vi "Measurement selected.vi"(8 "error in (no error)":errorcluster, 10 "Coords":T1, 11 "ZenGage v3.0 UI in":T2) -> (0 "error out":errorcluster, 3 "ZenGage v3.0 UI in":T2)   [LabVIEW 2019, in "ZenGage v3.0 UI.lvclass"]
uses:
  ZenGage v3.0 UI.lvclass
  <vilib>/Utility/miscctls.llb/LVPoint32TypeDef.ctl
  Type Definitions/JSON Read/UI JSON read cluster.ctl
  Type Definitions/General/JSONRead.ctl
  Type Definitions/Inspection/Inspection Cluster.ctl
  Type Definitions/Diagnostics/Diagnostics(Cluster).ctl
  Type Definitions/Edit tolerance settings/Rack Selection.ctl
  Type Definitions/Edit tolerance settings/Edit Tolerance Input.ctl
  Type Definitions/Edit tolerance settings/Edit Tolerance Overall Cluster.ctl
  Type Definitions/Controls and Indicators/Select a part (combobox).ctl
  Type Definitions/Controls and Indicators/EDL control references.ctl
  Type Definitions/Controls and Indicators/Diagnostics control referencs.ctl
  Type Definitions/Controls and Indicators/Inspection control references.ctl
  Type Definitions/Controls and Indicators/General_Control references.ctl
  Type Definitions/Controls and Indicators/Controls and Indicators Cluster.ctl
  Common/Controls/Pop-up Input.ctl
  Type Definitions/General/UI States(UI button enable disable).ctl
  Type Definitions/General/UIDataCluster.ctl
  Type Definitions/General/Master sample references.ctl
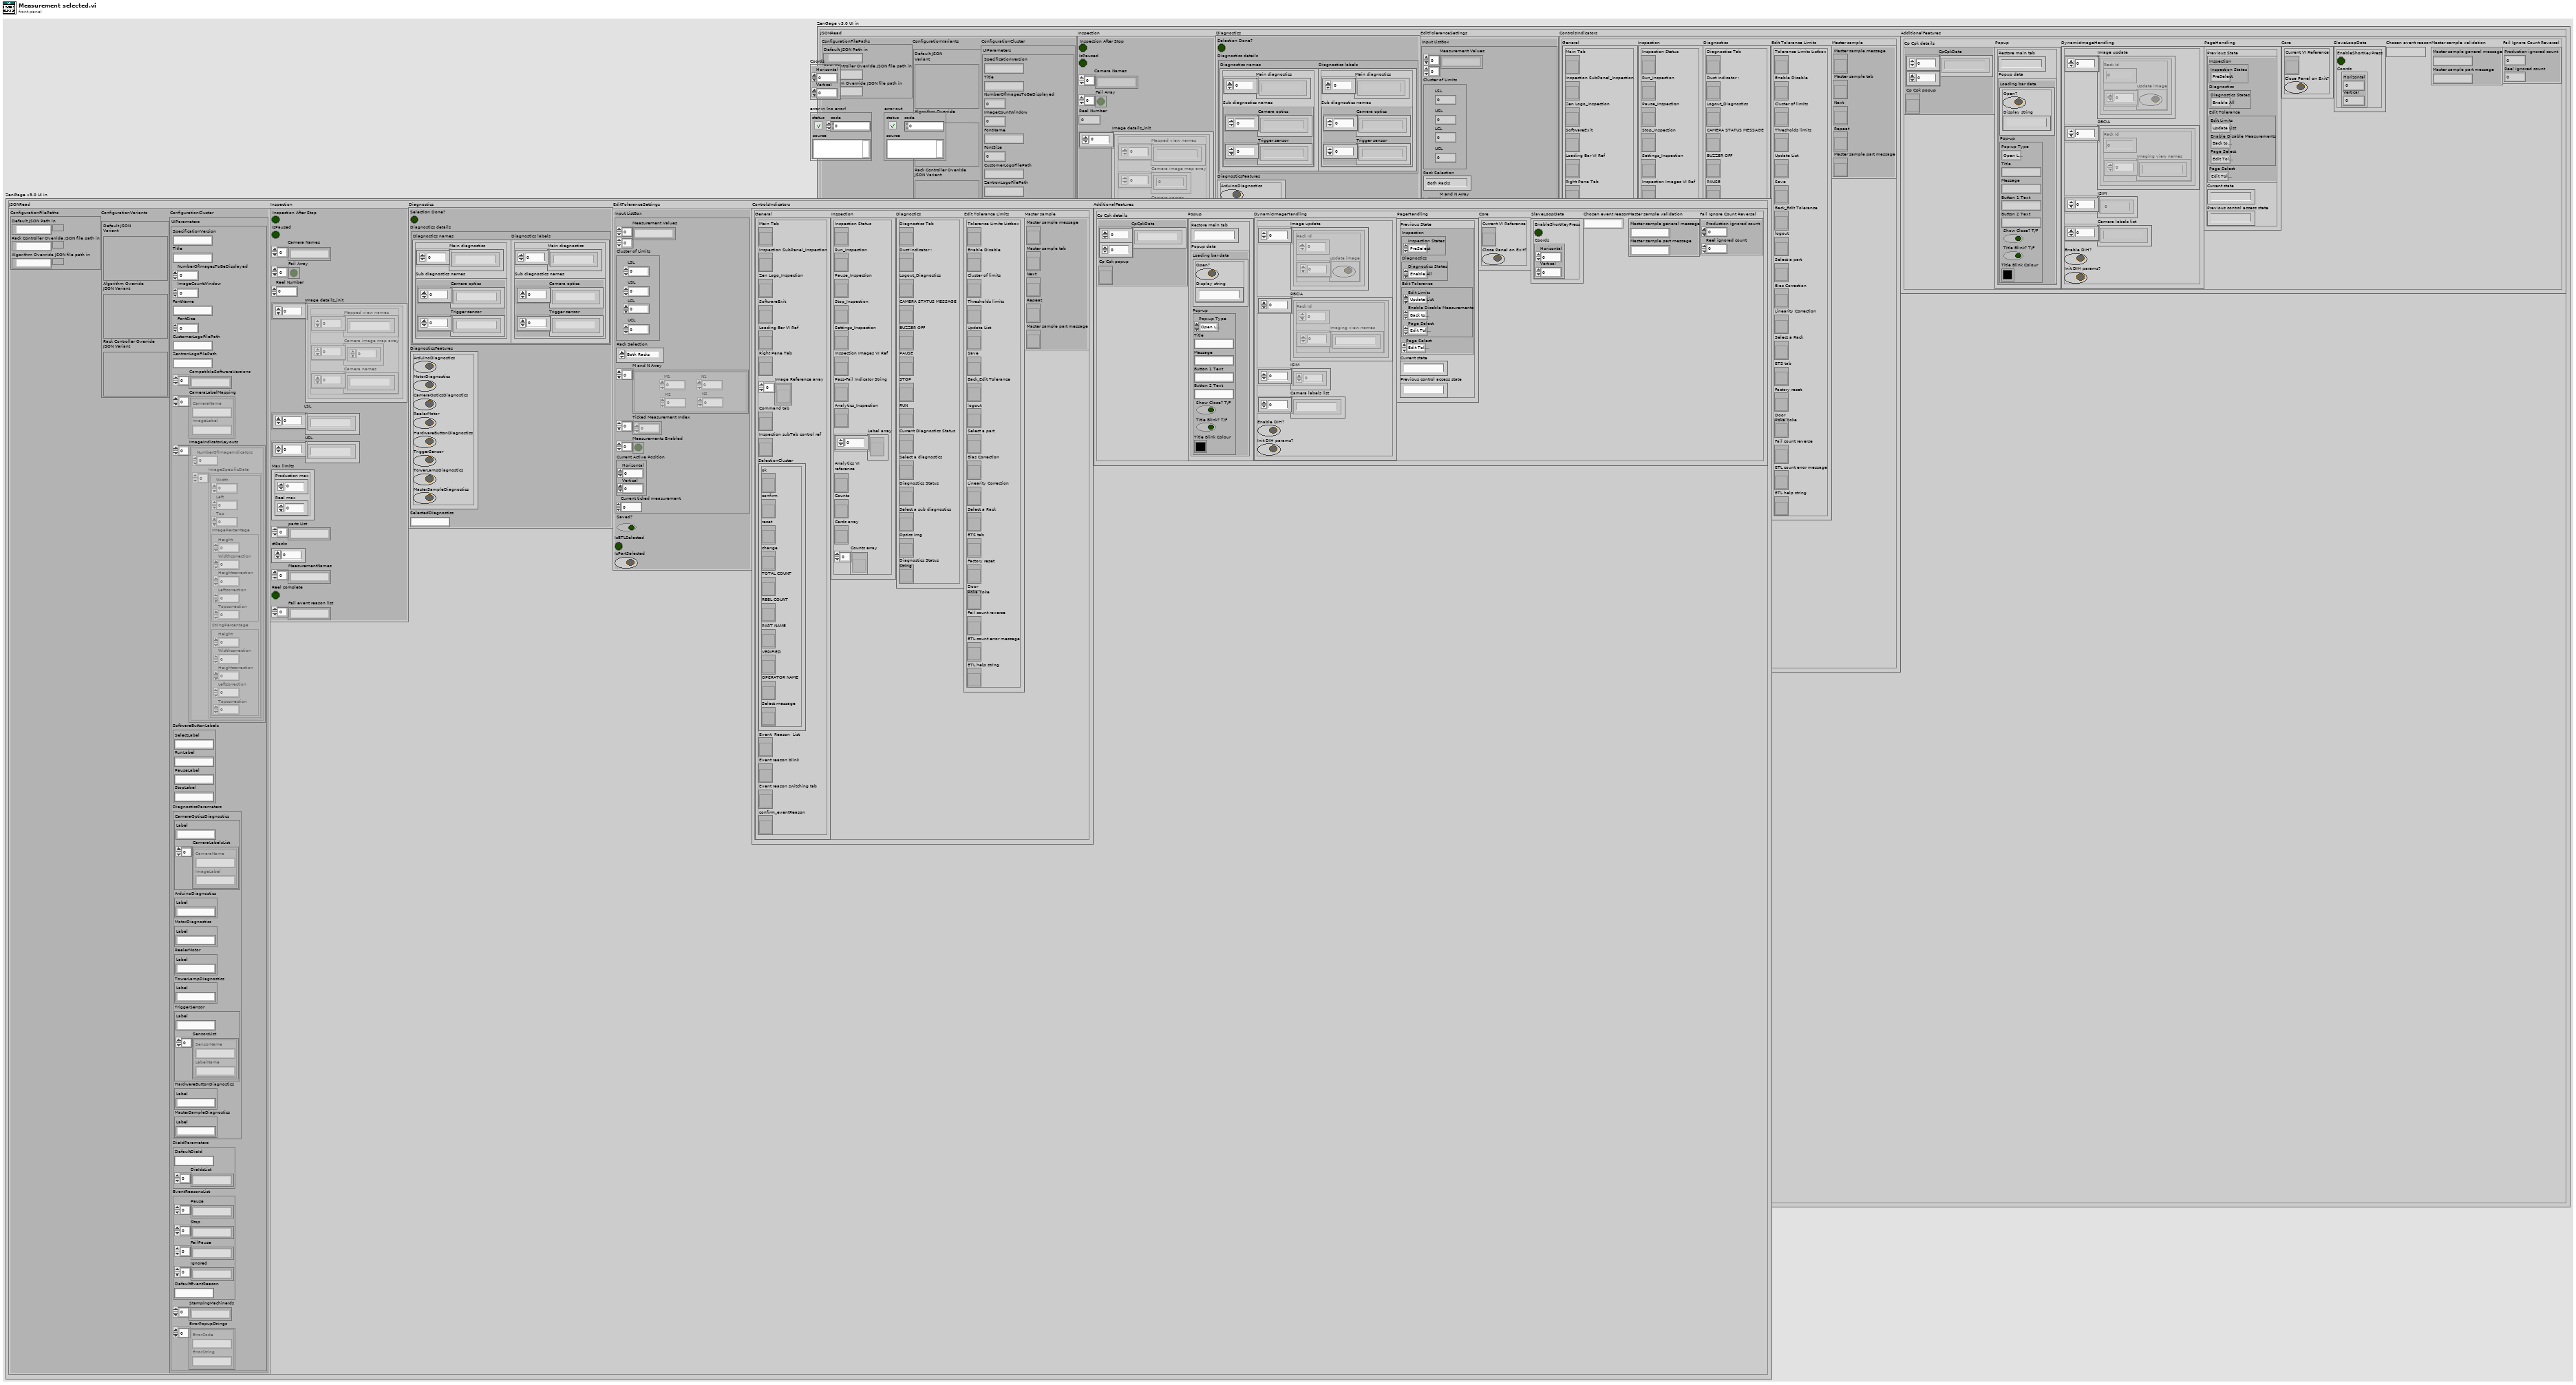
[diagram p1: front panel]
types:
  T1 = typedef "LVPoint32TypeDef.ctl" = cluster{"Horizontal":i32, "Vertical":i32}
  T2 = typedef "UIDataCluster.ctl" = cluster{"JSONRead":T3, "Inspection":T5, "Diagnostics":T6, "EditToleranceSettings":T7, "ControlsIndicators":T10, "AdditionalFeatures":cluster{"Cp Cpk details":cluster{"CpCpkData":string[][], "Cp Cpk popup":refnum<vi>}, "Popup":cluster{"Restore main tab":string, "Popup data":cluster{"Loading bar data":cluster{"Open?":bool, "Display string":string}, "Pop-up":T16}}, "DynamicImageHandling":cluster{"Image update":cluster{"Rack Id":i32, "Update image":bool[]}[], "RBCIA":cluster{"Rack Id":u8, "Imaging view names":string[]}[], "ISIM":u8[], "Camera labels list":string[], "Enable DIH?":bool, "Init DIH params?":bool}, "PageHandling":cluster{"Previous State":T17, "Current state":string, "Previous control access state":string}, "Core":cluster{"Current VI Reference":refnum<vi>, "Close Panel on Exit?":bool}, "SlaveLoopData":cluster{"EnableShortKeyPress":bool, "Point32":T1}, "Chosen event reason":string, "Master sample validation":cluster{"Master sample general message":string, "Master sample part message":string}, "Fail Ignore Count Reversal":cluster{"Production ignored count":u64, "Reel ignored count":u64}}}
  T3 = typedef "ZenGage v3.0 UI.lvclass/JSONRead.ctl" = cluster{"ConfigurationFilePaths":cluster{"Default JSON Path in":path, "Rack Controller Override JSON file path in":path, "Algorithm Overrride JSON file path in ":path}, "ConfigurationVariants":cluster{"Default JSON \nVariant":variant, "Algorithm Override\nJSON Variant":variant, "Rack Controller Override\nJSON Variant":variant}, "ConfigurationCluster":T4}
  T4 = typedef "ZenGage v3.0 UI.lvclass/UI JSON read cluster.ctl" = cluster{"UIParameters":cluster{"SpecificationVersion":string, "Title":string, "NumberOfImagesToBeDisplayed":dbl, "ImageCountWindow":dbl, "FontName":string, "FontSize":dbl, "CustomerLogoFilePath":string, "ZentronLogoFilePath":string, "CompatibleSoftwareVersions":string[], "CameraLabelMapping":cluster{"CameraName":string, "ImageLabel":string}[], "ImageIndicatorLayouts":cluster{"NumberOfImageIndicators":dbl, "ImageSpecificData":cluster{"Width":dbl, "Left":dbl, "Top":dbl, "ImagePercentage":cluster{"Height":dbl, "Widthcorrection":i64, "Heightcorrection":i64, "Leftcorrection":dbl, "Topcorrection":dbl}, "StringPercentage":cluster{"Height":dbl, "Widthcorrection":i64, "Heightcorrection":dbl, "Leftcorrection":dbl, "Topcorrection":dbl}}[]}[], "SoftwareButtonLabels":cluster{"SelectLabel":string, "RunLabel":string, "PauseLabel":string, "StopLabel":string}, "DiagnosticsParameters":cluster{"CameraOpticsDiagnostics":cluster{"Label":string, "CameraLabelsList":cluster{"CameraName":string, "ImageLabel":string}[]}, "ArduinoDiagnostics":cluster{"Label":string}, "MotorDiagnostics":cluster{"Label":string}, "ReelerMotor":cluster{"Label":string}, "TowerLampDiagnostics":cluster{"Label":string}, "TriggerSensor":cluster{"Label":string, "SensorsList":cluster{"SensorName":string, "LabelName":string}[]}, "HardwareButtonDiagnostics":cluster{"Label":string}, "MasterSampleDiagnostics":cluster{"Label":string}}, "DieIdParameters":cluster{"DefaultDieId":string, "DieIdsList":string[]}, "EventReasonsList":cluster{"Pause":string[], "Stop":string[], "FailPause":string[], "Ignored":string[], "DefaultEventReason":string}, "StampingMachineIds":string[], "ErrorPopupStrings":cluster{"ErrorCode":string, "ErrorString":string}[]}}
  T5 = typedef "ZenGage v3.0 UI.lvclass/Inspection Cluster.ctl" = cluster{"Inspection After Stop":bool, "IsPaused":bool, "Camera Names":string[], "Fail Array":bool[], "Reel Number":u32, "Image details_init":cluster{"Mapped view names":string[], "Camera image map array":i32[], "Camera names":string[]}[], "LSL":string[], "USL":string[], "Max limits":cluster{"Production max":u64, "Reel max":u64}, "parts List":string[], "#Racks":u8, "MeasurementNames":string[], "Reel complete":bool, "Fail event reason list":string[]}
  T6 = typedef "ZenGage v3.0 UI.lvclass/Diagnostics(Cluster).ctl" = cluster{"Selection Done?":bool, "Diagnostics details":cluster{"Diagnostics names":cluster{"Main diagnostics":string[], "Sub diagnostics names":cluster{"Camera optics":string[], "Trigger sensor":string[]}}, "Diagnostics labels":cluster{"Main diagnostics":string[], "Sub diagnostics names":cluster{"Camera optics":string[], "Trigger sensor":string[]}}}, "DiagnosticsFeatures":cluster{"ArduinoDiagnostics":bool, "MotorDiagnostics":bool, "CameraOpticsDiagnostics":bool, "ReelerMotor":bool, "HardwareButtonDiagnostics":bool, "TriggerSensor":bool, "TowerLampDiagnostics":bool, "MasterSampleDiagnostics":bool}, "SelectedDiagnostics":string}
  T7 = typedef "ZenGage v3.0 UI.lvclass/Edit Tolerance Overall Cluster.ctl" = cluster{"Input ListBox":T8, "Saved?":bool, "IsETLSelected":bool, "IsPartSelected":bool}
  T8 = typedef "ZenGage v3.0 UI.lvclass/Edit Tolerance Input.ctl" = cluster{"Measurement Values":string[][], "Cluster of Limits":cluster{"LSL":dbl, "USL":dbl, "LCL":dbl, "UCL":dbl}, "Rack Selection":T9, "M and N Array":cluster{"M1":u64, "M2":u64, "N1":u64, "N2":u64}[], "Ticked Measurement Index":u32[], "Measurements Enabled":bool[], "Current Active Position":T1, "Current ticked measurement":dbl}
  T9 = typedef "ZenGage v3.0 UI.lvclass/Rack Selection.ctl" = enum16{"Both Racks", "Rack 2", "Rack 1"}
  T10 = typedef "ZenGage v3.0 UI.lvclass/Controls and Indicators Cluster.ctl" = cluster{"General":T11, "Inspection":T12, "Diagnostics":T13, "Edit Tolerance Limits":T14, "Master sample":T15}
  T11 = typedef "ZenGage v3.0 UI.lvclass/General_Control references.ctl" = cluster{"Main Tab":refnum<vi>, "Inspection SubPanel_Inspection":refnum<vi>, "Zen Logo_Inspection":refnum<vi>, "SoftwareExit":refnum<vi>, "Loading Bar VI Ref":refnum<vi>, "Right Pane Tab":refnum<vi>, "Image Reference array":refnum<vi>[], "Command tab":refnum<vi>, "Inspection subTab control ref":refnum<vi>, "SelectionCluster":cluster{"ok":refnum<vi>, "confirm":refnum<vi>, "reset":refnum<vi>, "change":refnum<vi>, "TOTAL COUNT":refnum<vi>, "REEL COUNT":refnum<vi>, "PART NAME":refnum<vi>, "VERIFIED":refnum<vi>, "OPERATOR NAME":refnum<vi>, "Select message":refnum<vi>}, "Event  Reason  List":refnum<vi>, "Event reason blink":refnum<vi>, "Event reason switching tab":refnum<vi>, "confirm_eventReason":refnum<vi>}
  T12 = typedef "ZenGage v3.0 UI.lvclass/Inspection control references.ctl" = cluster{"Inspection Status":refnum<vi>, "Run_Inspection":refnum<vi>, "Pause_Inspection":refnum<vi>, "Stop_Inspection":refnum<vi>, "Settings_Inspection":refnum<vi>, "Inspection Images VI Ref":refnum<vi>, "Pass-Fail Indicator String":refnum<vi>, "Analytics_Inspection":refnum<vi>, "Label array":refnum<vi>[], "Analytics VI\nreference":refnum<vi>, "Counts":refnum<vi>, "Cards array":refnum<vi>, "Counts array":refnum<vi>[]}
  T13 = typedef "ZenGage v3.0 UI.lvclass/Diagnostics control referencs.ctl" = cluster{"Diagnostics Tab":refnum<vi>, "Dust indicator :":refnum<vi>, "Logout_Diagnostics":refnum<vi>, "CAMERA STATUS MESSAGE":refnum<vi>, "BUZZER OFF":refnum<vi>, "PAUSE":refnum<vi>, "STOP":refnum<vi>, "RUN":refnum<vi>, "Current Diagnostics Status":refnum<vi>, "Select a diagnostics":refnum<vi>, "Diagnostics Status":refnum<vi>, "Select a sub diagnostics":refnum<vi>, "Optics img":refnum<vi>, "Diagnostics Status\nString":refnum<vi>}
  T14 = typedef "ZenGage v3.0 UI.lvclass/EDL control references.ctl" = cluster{"Tolerance Limits Listbox":refnum<vi>, "Enable Disable":refnum<vi>, "Cluster of limits":refnum<vi>, "Thresholds limits":refnum<vi>, "Update List":refnum<vi>, "Save":refnum<vi>, "Back_Edit Tolerance":refnum<vi>, "logout":refnum<vi>, "Select a part":refnum<vi>, "Bias Correction":refnum<vi>, "Linearity Correction":refnum<vi>, "Select a Rack":refnum<vi>, "ETS tab":refnum<vi>, "Factory reset":refnum<vi>, "Door\nPoka Yoke":refnum<vi>, "Fail count reverse":refnum<vi>, "ETL count error message":refnum<vi>, "ETL help string":refnum<vi>}
  T15 = typedef "Master sample references.ctl" = cluster{"Master sample message":refnum<vi>, "Master sample tab":refnum<vi>, "Next":refnum<vi>, "Repeat":refnum<vi>, "Master sample part message":refnum<vi>}
  T16 = typedef "Pop-up Input.ctl" = cluster{"Pop-up Type":enum16{"Open Logo Display", "Close Logo Display", "Open Loading Bar", "Close Loading Bar", "Open Alert Display", "Close Alert Display", "One button dialog box", "Two button dialog box", "User Authentication"}, "Title":string, "Message":string, "Button 1 Text":string, "Button 2 Text":string, "Show Close? T/F":bool, "Title Blink? T/F":bool, "Title Blink Colour":u32}
  T17 = typedef "ZenGage v3.0 UI.lvclass/UI States(UI button enable disable).ctl" = cluster{"Inspection":cluster{"Inspection States":enum16{"PreSelect", "Back _Inspection", "Analytics", "Ready To Run", "Ready To Insert", "Enable All buttons", "Disable All Buttons", "Settings", "Select", "Stop", "Pause", "Inspect"}}, "Diagnostics":cluster{"Diagnostics States":enum16{"Enable All", "Camera Optics Fail", "Loading Bar", "Camera Optics", "Motor", "Arduino", "POST Done", "POST"}}, "Edit Tolerance":cluster{"Edit Limits":enum16{"Update List"}, "Enable Disable Measurements":enum16{"Back to Edit Tolerance"}, "Page Select":enum16{"Edit Tolerance Limits", "Enable Disable Buttons"}}, "Page Select":enum16{"Edit Tolerance", "Diagnostics", "Inspection"}}
  T18 = cluster{"Ticked Measurement Index":u32[], "M and N array":cluster{"M1":u64, "M2":u64, "N1":u64, "N2":u64}[], "Current ticked measurement":dbl, "Current Active Position":T1}
  T19 = cluster{"Cluster of limits":refnum<vi>, "Linearity correction":refnum<vi>, "Bias correction":refnum<vi>, "ToleranceLimitsListbox":refnum<vi>}
  T20 = enum8{"Enabled", "Disabled", "Disabled and Grayed Out"}
  T21 = cluster{"M1":u64, "M2":u64, "N1":u64, "N2":u64}[]
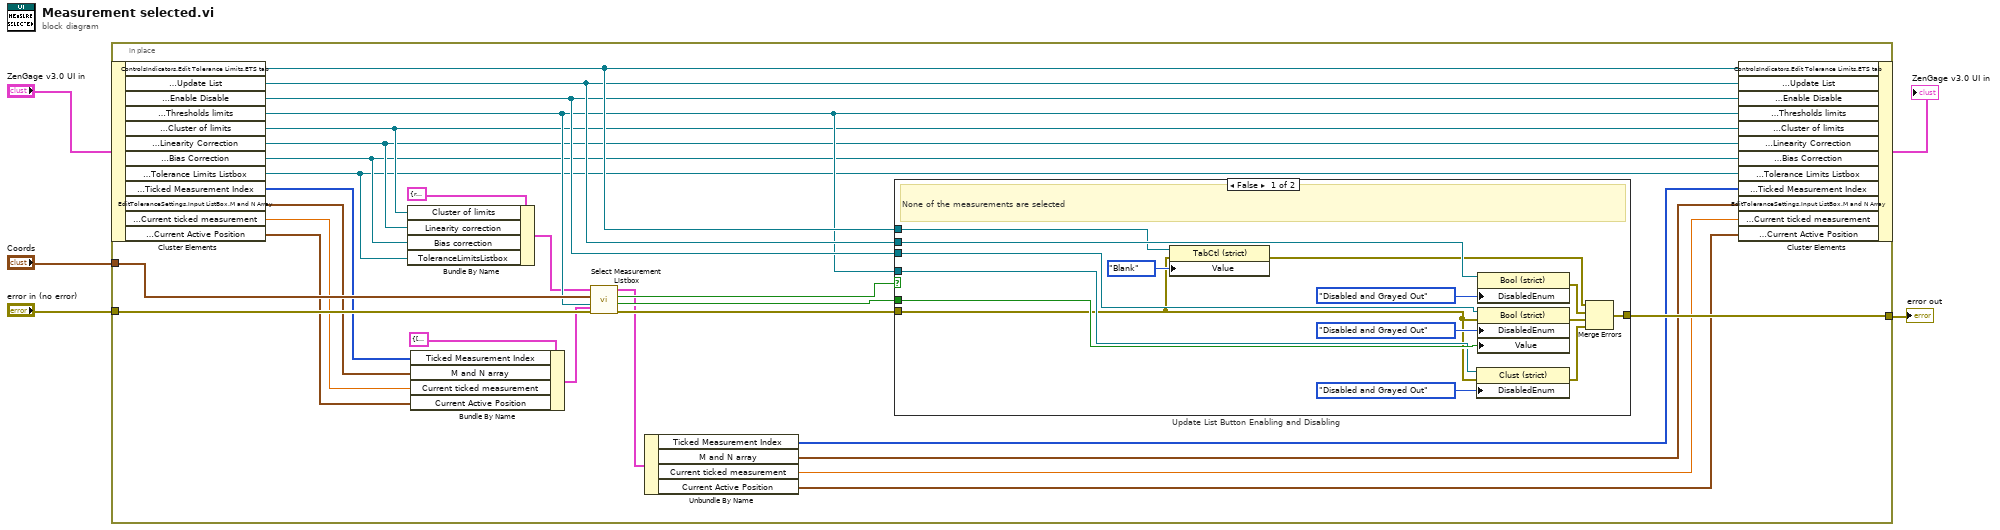
[diagram p0: block diagram]
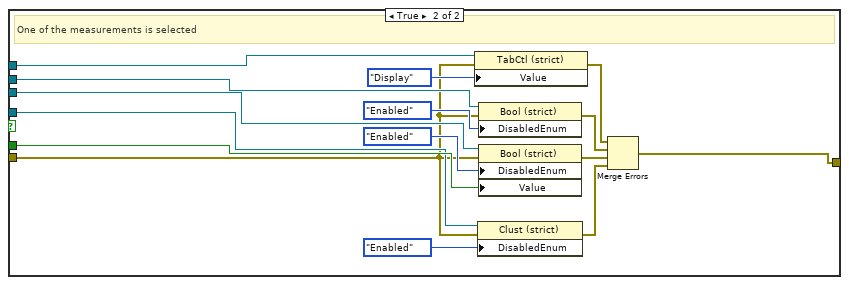
[diagram p2: hidden frame]
diagram:
  n1 = in-place {
    in-place-border: "Coords" -> [w29]
    in-place-border: "error in (no error)" -> [w28]
    in-place-border: [w24] -> w2
    n2 = in-place-cluster #1("ZenGage v3.0 UI in") -> ("ControlsIndicators.Edit Tolerance Limits.ETS tab"=w27:refnum<vi>, "ControlsIndicators.Edit Tolerance Limits.Update List"=w26:refnum<vi>, "ControlsIndicators.Edit Tolerance Limits.Enable Disable"=w25:refnum<vi>, "ControlsIndicators.Edit Tolerance Limits.Thresholds limits"=w23:refnum<vi>, "ControlsIndicators.Edit Tolerance Limits.Cluster of limits"=w21:refnum<vi>, "ControlsIndicators.Edit Tolerance Limits.Linearity Correction"=w20:refnum<vi>, "ControlsIndicators.Edit Tolerance Limits.Bias Correction"=w19:refnum<vi>, "ControlsIndicators.Edit Tolerance Limits.Tolerance Limits Listbox"=w18:refnum<vi>, "EditToleranceSettings.Input ListBox.Ticked Measurement Index"=w14:u32[], "EditToleranceSettings.Input ListBox.M and N Array"=w7:T21, "EditToleranceSettings.Input ListBox.Current ticked measurement"=w6:dbl, "EditToleranceSettings.Input ListBox.Current Active Position"=w13:T1)
    n3 = Bundle By Name(cluster=T19 {"Cluster of limits"=refnum, "Linearity correction"=refnum, "Bias correction"=refnum, "ToleranceLimitsListbox"=refnum} ("References in"), "Cluster of limits"=w21, "Linearity correction"=w20, "Bias correction"=w19, "ToleranceLimitsListbox"=w18) -> (w17:T19)
    n4 = Bundle By Name(cluster=T18 {"Ticked Measurement Index"=[], "M and N array"=[], "Current ticked measurement"=0.0, "Current Active Position"={"Horizontal"=0, "Vertical"=0}} ("Cluster in"), "Ticked Measurement Index"=w14, "M and N array"=w7, "Current ticked measurement"=w6, "Current Active Position"=w13) -> (w15:T18)
    n5 = call "Select Measurement Listbox.vi"("Cluster in"=w15, "error in (no error)"=w28, "ThresholdLimits"=w23, "Coords"=w29, "References in"=w17) -> ("error out"=w30:errorcluster, "Enable Disable button state"=w32:bool, "Tick Marked?"=w31:bool, "Cluster out"=w12:T18)  [unwired: 3 in]
    n6 = Unbundle By Name(w12) -> ("Ticked Measurement Index"=w11:u32[], "M and N array"=w10:T21, "Current ticked measurement"=w9:dbl, "Current Active Position"=w8:T1)
    n7 = case "Update List Button Enabling and Disabling" shown="False" w31 {
      tunnel: w26 -> [w47 w62]
      tunnel: [w42 w57] -> w24
      tunnel: w32 -> [w41 w56]
      tunnel: w30 -> [w33 w48]
      tunnel: w25 -> [w40 w55]
      tunnel: w23 -> [w39 w53]
      tunnel: w27 -> [w36 w50]
      frame False {
        # "None of the measurements are selected"
        n8 = property class="TabCtl (strict)"(reference=w36, error in=w33, "Value"=enum32{"Display", "Blank"}."Blank") -> (error out=w34:errorcluster)  [unwired: 1 out]
        n9 = property class="Clust (strict)"(reference=w39, error in=w33, "DisabledEnum"=T20."Disabled and Grayed Out" ("Disabled")) -> (error out=w38:errorcluster)  [unwired: 1 out]
        n10 = property class="Bool (strict)"(reference=w47, "DisabledEnum"=T20."Disabled and Grayed Out" ("Disabled")) -> (error out=w43:errorcluster)  [unwired: 1 in, 1 out]
        n11 = property class="Bool (strict)"(reference=w40, error in=w33, "DisabledEnum"=T20."Disabled and Grayed Out" ("Disabled"), "Value"=w41) -> (error out=w44:errorcluster)  [unwired: 1 out]
        n12 = Merge Errors(w34, w43, w44, w38) -> (w42:errorcluster)
      }
      frame True {
        # "One of the measurements is selected"
        n13 = property class="TabCtl (strict)"(reference=w50, error in=w48, "Value"=enum32{"Display", "Blank"}."Display") -> (error out=w51:errorcluster)  [unwired: 1 out]
        n14 = property class="Clust (strict)"(reference=w53, error in=w48, "DisabledEnum"=T20."Enabled" ("Disabled")) -> (error out=w54:errorcluster)  [unwired: 1 out]
        n15 = property class="Bool (strict)"(reference=w62, error in=w48, "DisabledEnum"=T20."Enabled" ("Disabled")) -> (error out=w58:errorcluster)  [unwired: 1 out]
        n16 = property class="Bool (strict)"(reference=w55, error in=w48, "DisabledEnum"=T20."Enabled" ("Disabled"), "Value"=w56) -> (error out=w59:errorcluster)  [unwired: 1 out]
        n17 = Merge Errors(w51, w58, w59, w54) -> (w57:errorcluster)
      }
    }
    n18 = in-place-cluster #1("ControlsIndicators.Edit Tolerance Limits.ETS tab"=w27, "ControlsIndicators.Edit Tolerance Limits.Update List"=w26, "ControlsIndicators.Edit Tolerance Limits.Enable Disable"=w25, "ControlsIndicators.Edit Tolerance Limits.Thresholds limits"=w23, "ControlsIndicators.Edit Tolerance Limits.Cluster of limits"=w21, "ControlsIndicators.Edit Tolerance Limits.Linearity Correction"=w20, "ControlsIndicators.Edit Tolerance Limits.Bias Correction"=w19, "ControlsIndicators.Edit Tolerance Limits.Tolerance Limits Listbox"=w18, "EditToleranceSettings.Input ListBox.Ticked Measurement Index"=w11, "EditToleranceSettings.Input ListBox.M and N Array"=w10, "EditToleranceSettings.Input ListBox.Current ticked measurement"=w9, "EditToleranceSettings.Input ListBox.Current Active Position"=w8) -> (→"ZenGage v3.0 UI in":T2)
  }
  "error out" <- w2
